vi "Write.vi"(8 "error in (no error)":errorcluster, 10 "PV":refnum<class "PV.lvclass">, 11 "PVConnection in":refnum<class "SVConnection.lvclass">) -> (0 "error out":errorcluster, 3 "PVConnection out":refnum<class "SVConnection.lvclass">)   [LabVIEW 2013, in "CS++ProcessVariables.lvlib" / "SVConnection.lvclass"]
doc: "Publish a process varibale."
uses:
  SVConnection.lvclass
  ProcessVariable/PV.lvclass
  SVConnection.lvclass/SVConnection.ctl
  ProcessVariable/PV.lvclass/PV.ctl
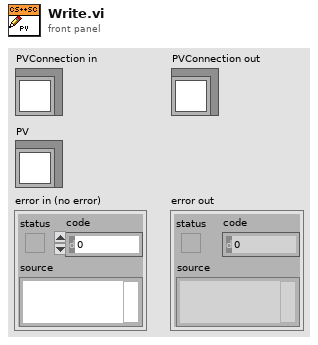
[diagram p1: front panel]
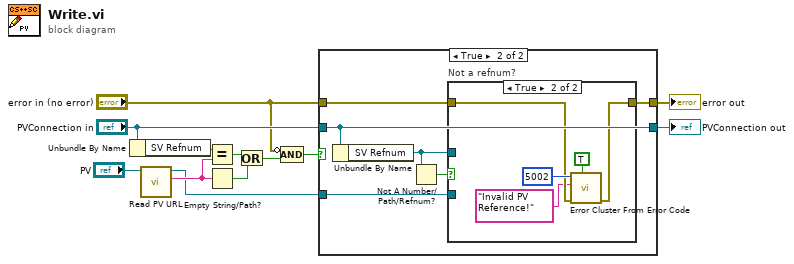
[diagram p0: block diagram]
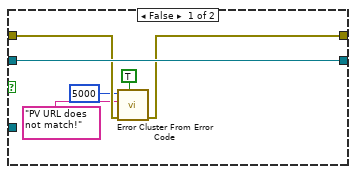
[diagram p2: hidden frame]
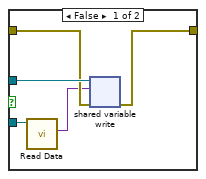
[diagram p3: hidden frame]
diagram:
  n1 = Unbundle By Name("PVConnection in") -> ("SV Refnum"=w7:refnum<k21>)
  n2 = call "Read PV URL.vi"("PV in"="PV") -> ("PV URL"=w6:string, "PV out"=w1:refnum<class "PV.lvclass">)  [unwired: 8 in, 1 out]
  n3 = Equal?(x=w7, y=w6) -> (x = y?=w5:bool)
  n4 = Empty String/Path?(string/path=w6) -> (empty?=w9:bool)
  n5 = Or(x=w5, y=w9) -> (x .or. y?=w4:bool)
  n6 = Compound Arithmetic op=AND(invert "error in (no error)", w4) -> (w3:bool)
  n7 = case shown="True" w3 {
    tunnel: [w16 w22] -> w12
    tunnel: [w18 w24] -> w11
    tunnel: "PVConnection in" -> [w18 w24]
    tunnel: "error in (no error)" -> [w17 w23]
    tunnel: w1 -> [_ w21]
    frame False {
      n8 = call <vilib>:"Error Cluster From Error Code.vi"("show call chain? (False)"=TRUE, "error in (no error)"=w17, "error message (\"\")"="PV URL does not match!" ("error message (\"\")"), "error code (0)"=5000) -> ("error out"=w16:errorcluster)  [unwired: 5 in]
    }
    frame True {
      n9 = Unbundle By Name(w24) -> ("SV Refnum"=w19:refnum<k21>)
      n10 = Not A Number/Path/Refnum?(number/path/refnum=w19) -> (NaN/Path/Refnum?=w20:bool)
      n11 = case "Not a refnum?" shown="True" w20 {
        tunnel: w19 -> [w29 _]
        tunnel: w23 -> [w28 w32]
        tunnel: [w27 w31] -> w22
        tunnel: w21 -> [w25 _]
        frame False {
          n12 = call "Read Data.vi"("PV in"=w25) -> ("Data"=w26:variant)  [unwired: 8 in, 2 out]
          n13 = shared-variable-write(w29, w28, w26) -> (w27:errorcluster)  [unwired: 1 out]
        }
        frame True {
          n14 = call <vilib>:"Error Cluster From Error Code.vi"("show call chain? (False)"=TRUE, "error in (no error)"=w32, "error message (\"\")"="Invalid PV Reference!" ("error message (\"\")"), "error code (0)"=5002) -> ("error out"=w31:errorcluster)  [unwired: 5 in]
        }
      }
    }
  }
  "error out" <- w12
  "PVConnection out" <- w11
